vi "Generate CSV File & Path with Headings.vi"(8 "Heading 2":string, 9 "Heading 1":string, 10 "Relative Path or Folder":path, 11 "File Name":string) -> (0 "error out":errorcluster, 1 "Log Date & Time":string, 2 "Log File Path":path, 3 "Byte Stream File out":refnum<file>, 5 "Log File Name":string)   [LabVIEW 2021]
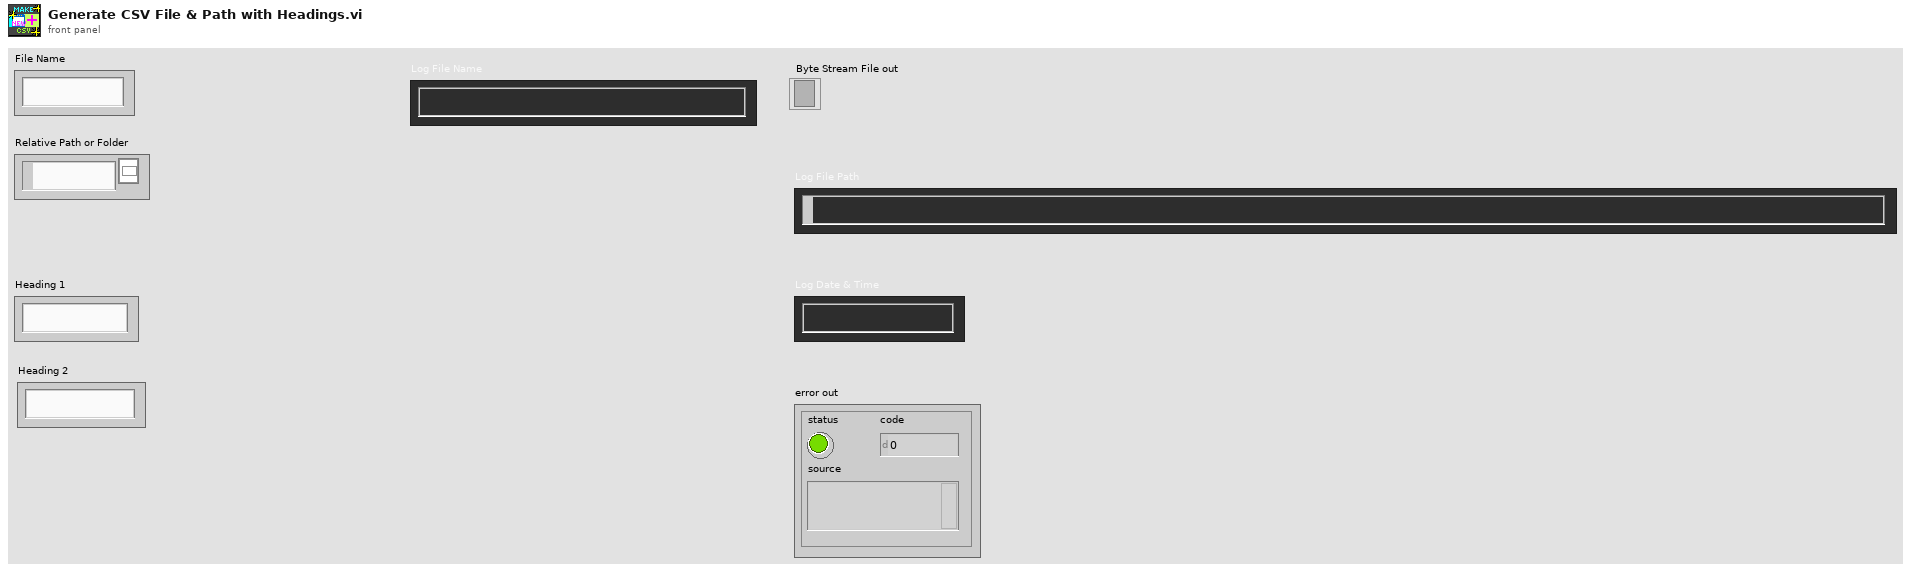
[diagram p1: front panel]
types:
  T1 = enum16{"open", "replace", "create", "open or create", "replace or create", "replace or create with confirmation"}
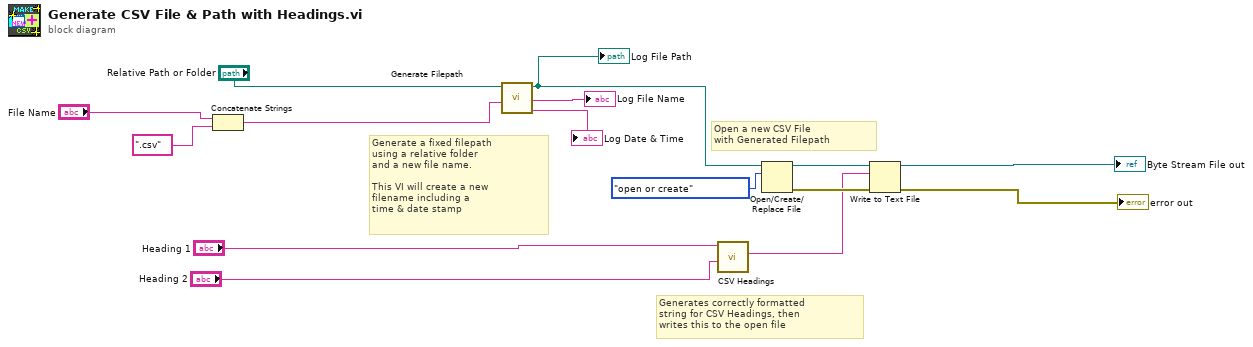
[diagram p0: block diagram]
diagram:
  # "Generates correctly formatted\nstring for CSV Headings, then\nwrites this to the open file"
  # "Open a new CSV File\nwith Generated Filepath"
  # "Generate a fixed filepath\nusing a relative folder\nand a new file name.\n\nThis VI will create a new\nfilename including a\ntime & date stamp"
  n1 = Concatenate Strings("File Name", ".csv" ("string")) -> (w2:string)
  n2 = call "Generate Filepath.vi"("File Name"=w2, "Relative Path or Folder"="Relative Path or Folder") -> ("Date & Time"=→"Log Date & Time":string, "Log File Name"=→"Log File Name":string, "File Path Output"=w6:path)  [unwired: 7 in]
  "Log File Path" <- w6
  n3 = call "CSV Headings.vi"("Heading 2"="Heading 2", "Heading 1"="Heading 1") -> ("CSV Heading String"=w11:string)  [unwired: 9 in]
  n4 = Open/Create/Replace File(file path (use dialog)=w6, operation (0:open)=T1."open or create") -> (refnum out=w7:refnum<file>, error out=w15:errorcluster)  [unwired: 4 in, 1 out]
  n5 = Write to Text File(file (use dialog)=w7, text=w11, error in=w15) -> (refnum out=→"Byte Stream File out":refnum<file>, error out=→"error out":errorcluster)  [unwired: 1 in, 1 out]
